vi "Destroy Broadcast Events.vi"(8 "error in":errorcluster) -> (0 "error out":errorcluster)   [LabVIEW 2026, in "Acquisition.lvlib"]
doc: "Destroy the broadcast events, even if there is an incoming error.\n\n<b>NOTE</b>: The contents of this VI are automatically generated and modified by the <b>Tools > DQMH Consortium > DQMH</b> utilities. Consider using those utilities instead of making your own modifications to this VI.\n_____\nBased on DQMH Project Template 4.0.0.47.\n_____\nBased on DQMH Dev Tools: Project Template 7.1.2.1547."
uses:
  Acquisition.lvlib
panel:
  # "NOTE: The contents of this VI are automatically generated and modified by the Tools > DQMH Consortium > DQMH utilities. Consider using those utilities instead of making your own modifications to this VI."
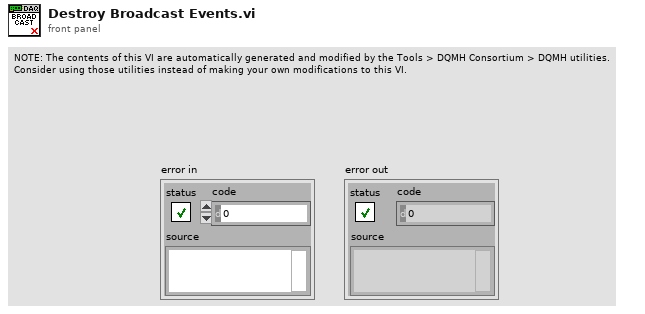
[diagram p1: front panel]
types:
  T1 = typedef "Acquisition.lvlib/Broadcast Events--cluster.ctl" = cluster{"Module Did Init":refnum<user-event>, "Status Updated":refnum<user-event>, "Error Reported":refnum<user-event>, "Module Did Stop":refnum<user-event>, "Update Module Execution Status":refnum<user-event>, "Acquisition Started":refnum<user-event>, "Acquisition Stopped":refnum<user-event>, "Data Updated":refnum<user-event>, "Device Calibrated":refnum<user-event>}
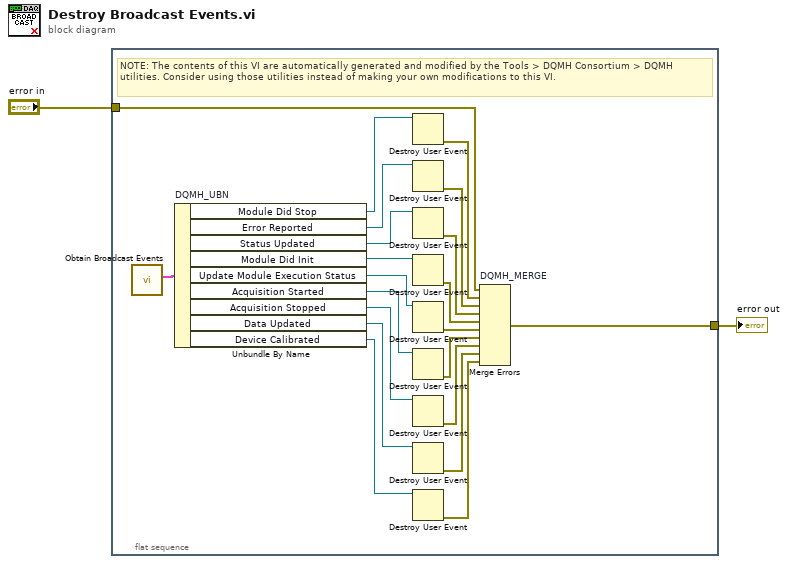
[diagram p0: block diagram]
diagram:
  n1 = flat-sequence {
    tunnel: [w22] -> w2
    tunnel: "error in" -> [w13]
    frame #0 {
      # "NOTE: The contents of this VI are automatically generated and modified by the Tools > DQMH Consortium > DQMH utilities. Consider using those utilities instead of making your own modifications to this VI."
      n2 = call "Obtain Broadcast Events.vi"() -> ("Acquisition Broadcast Events"=w21:T1)  [unwired: 10 in, 1 out]
      n3 = Unbundle By Name "DQMH_UBN"(w21) -> ("Module Did Stop"=w14:refnum<user-event>, "Error Reported"=w16:refnum<user-event>, "Status Updated"=w19:refnum<user-event>, "Module Did Init"=w20:refnum<user-event>, "Update Module Execution Status"=w11:refnum<user-event>, "Acquisition Started"=w9:refnum<user-event>, "Acquisition Stopped"=w7:refnum<user-event>, "Data Updated"=w5:refnum<user-event>, "Device Calibrated"=w3:refnum<user-event>)
      n4 = Destroy User Event(user event=w14) -> (error out=w15:errorcluster)  [unwired: 1 in]
      n5 = Destroy User Event(user event=w16) -> (error out=w17:errorcluster)  [unwired: 1 in]
      n6 = Destroy User Event(user event=w19) -> (error out=w18:errorcluster)  [unwired: 1 in]
      n7 = Destroy User Event(user event=w20) -> (error out=w23:errorcluster)  [unwired: 1 in]
      n8 = Destroy User Event(user event=w11) -> (error out=w12:errorcluster)  [unwired: 1 in]
      n9 = Destroy User Event(user event=w9) -> (error out=w10:errorcluster)  [unwired: 1 in]
      n10 = Destroy User Event(user event=w7) -> (error out=w8:errorcluster)  [unwired: 1 in]
      n11 = Destroy User Event(user event=w5) -> (error out=w6:errorcluster)  [unwired: 1 in]
      n12 = Destroy User Event(user event=w3) -> (error out=w4:errorcluster)  [unwired: 1 in]
      n13 = Merge Errors "DQMH_MERGE"(w13, w15, w17, w18, w23, w12, w10, w8, w6, w4) -> (w22:errorcluster)
    }
  }
  "error out" <- w2
